vi "Autonomous.vi"(11 "Call Context":T7) -> (0 "SubState 2":T2, 1 "Loop 2 Data":T3, 2 "SubState 1":T2, 3 "Loop 1 Data":T4, 4 "Loop 3 Data":T1, 5 "SubState 0":T2=enum."driver control", 6 "SubState 3":T2, 7 "Loop 0 Data":T5, 10 "SubState 4":T6)   [LabVIEW 2013]
uses:
  typedefs/State Machine/subStates.ctl
  <vilib>/Rock Robotics/WPI/DriverStation/WPI_DriverStationDerivedRobotMode.ctl
  typedefs/State Machine/singleUseSubstate.ctl
  typedefs/Loop Datatypes/Loop 0 Datatype.ctl
  typedefs/Loop Datatypes/Loop 1 Datatype.ctl
  typedefs/Loop Datatypes/Loop 2 Datatype.ctl
  typedefs/Loop Datatypes/Loop 3 Datatype.ctl
  typedefs/Vision/vision enable.ctl
  typedefs/fg_typedef.ctl
panel:
  # "Autonomous Loop Data"
  # "Robot Drive"
  # "State Machine Master"
  # "Pickup/Passing Belts"
  # "Pickup/Passing Arm"
  # "Pneumatics"
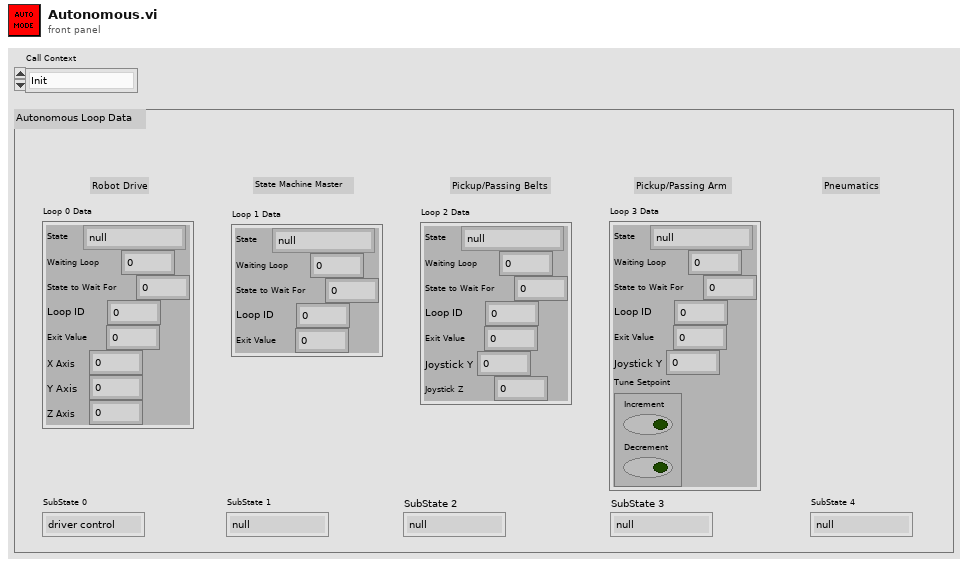
[diagram p1: front panel]
types:
  T1 = typedef "Loop 3 Datatype.ctl" = cluster{"State":T2, "Waiting Loop":i32, "State to Wait For":i32, "Loop ID":i32, "Exit Value":i32, "Joystick Y":dbl, "Tune Setpoint":cluster{"Increment":bool, "Decrement":bool}}
  T2 = typedef "subStates.ctl" = enum16{"null", "wait", "driver control", "auto", "manual override", "hold position", "rotate", "pickup", "pass", "recover pass", "load", "goto shoot", "shoot high goal", "shoot low goal", "cancel arm", "cancel shooter", "end", "test"}
  T3 = typedef "Loop 2 Datatype.ctl" = cluster{"State":T2, "Waiting Loop":i32, "State to Wait For":i32, "Loop ID":i32, "Exit Value":i32, "Joystick Y":dbl, "Joystick Z":dbl}
  T4 = typedef "Loop 1 Datatype.ctl" = cluster{"State":T2, "Waiting Loop":i32, "State to Wait For":i32, "Loop ID":i32, "Exit Value":i32}
  T5 = typedef "Loop 0 Datatype.ctl" = cluster{"State":T2, "Waiting Loop":i32, "State to Wait For":i32, "Loop ID":i32, "Exit Value":i32, "X Axis":dbl, "Y Axis":dbl, "Z Axis":dbl}
  T6 = typedef "singleUseSubstate.ctl" = enum16{"null", "wait", "shift high", "shift low", "extend shooter", "retract shooter", "latch", "unlatch", "end"}
  T7 = typedef "WPI_DriverStationDerivedRobotMode.ctl" = enum16{"Init", "Execute", "Stop"}
  T8 = typedef "fg_typedef.ctl" = enum16{"Get", "Set"}
  T9 = typedef "vision enable.ctl" = enum16{"Enable", "Disable", "Stop"}
  T10 = typedef "WPI_EncoderDevRef.ctl" = cluster{"DevStatus":errorcluster, "EncoderIndex":T11, "CounterIndex":T12, "DistancePerCount":dbl, "Decoding Type":T13}
  T11 = typedef "FPGA_EncoderIdx.ctl" = enum8{"Enc 0", "Enc 1", "Enc 2", "Enc 3", "Invalid"}
  T12 = typedef "FPGA_CounterCtrSystemIndex.ctl" = enum8{"Ctr 0", "Ctr 1", "Ctr 2", "Ctr 3", "Ctr 4", "Ctr 5", "Ctr 6", "Ctr 7", "Invalid"}
  T13 = typedef "WPI_EncoderType.ctl" = enum16{"1x", "2x", "4x"}
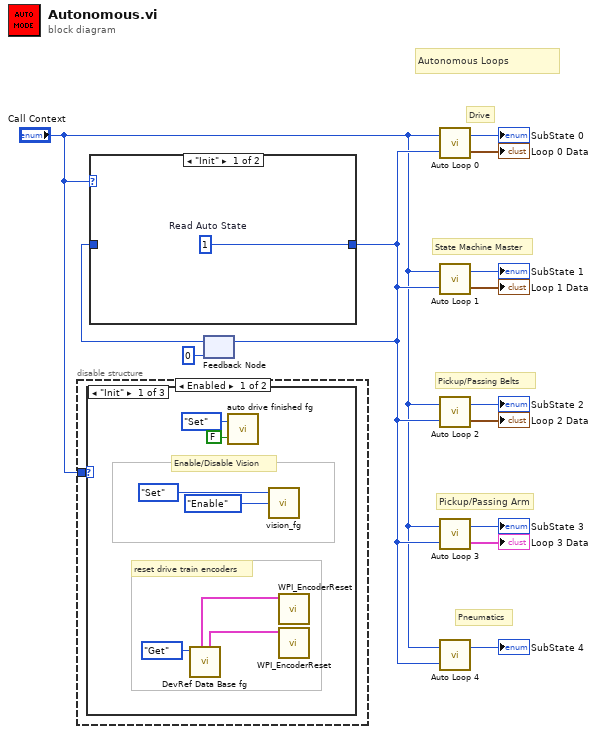
[diagram p0: block diagram]
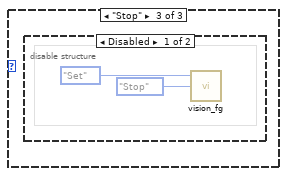
[diagram p3: hidden frame]
diagram:
  # "Autonomous Loops"
  # "Pickup/Passing Arm"
  # "Pickup/Passing Belts"
  # "Pneumatics"
  # "State Machine Master"
  # "Drive"
  n1 = disable-structure shown="Enabled" {
    disable-tunnel: "Call Context" -> [w14 _]
    frame Enabled {
      n2 = case shown="\"Init\"" w14 {
        frame "Init" {
          # "Enable/Disable Vision"
          # "reset drive train encoders"
          n3 = call "DevRef Data Base fg.vi"("Menu"=fg_typedef."Get") -> ("right drive encoder"=w17:T10, "left drive encoder"=w18:T10)  [unwired: 2 in, 7 out]
          n4 = call "auto drive finished fg.vi"("Done?"=FALSE, "Menu"=fg_typedef."Set") -> ()  [unwired: 1 out]
          n5 = call "vision_fg.vi"("Action"=vision_enable."Enable", "Menu"=fg_typedef."Set") -> ()  [unwired: 1 in, 2 out]
          n6 = call <vilib>:"WPI_EncoderReset.vi"("EncoderDevRef"=w18) -> ()  [unwired: 9 in, 2 out]
          n7 = call <vilib>:"WPI_EncoderReset.vi"("EncoderDevRef"=w17) -> ()  [unwired: 9 in, 2 out]
        }
        frame "Execute", Default {
        }
        frame "Stop" {
          n8 = disable-structure shown="Disabled" {
            frame Disabled {
              n9 = call "vision_fg.vi"("Action"=vision_enable."Stop", "Menu"=fg_typedef."Set") -> ()  [unwired: 1 in, 2 out]
            }
            frame Enabled {
            }
          }
        }
      }
    }
    frame Disabled {
    }
  }
  n10 = feedback #1(u8 0 ("Read Auto State")) -> (w2:u8)
  n11 = case shown="\"Init\"" "Call Context" {
    tunnel: [w24 w25] -> w4
    tunnel: w2 -> [_ w25]
    frame "Init" {
      w24 = u8 1  # Read Auto State
    }
    frame "Execute", Default {
    }
  }
  n12 = feedback-in #1(w4) -> ()
  n13 = call "Auto Loop 0.vi"("Auto State"=w4, "Call Context"="Call Context") -> ("Loop 0 Data"=→"Loop 0 Data":T5, "SubState 0"=→"SubState 0":T2)
  n14 = call "Auto Loop 1.vi"("Auto State"=w4, "Call Context"="Call Context") -> ("Loop 1 Data"=→"Loop 1 Data":T4, "SubState 1"=→"SubState 1":T2)
  n15 = call "Auto Loop 2.vi"("Auto State"=w4, "Call Context"="Call Context") -> ("Loop 2 Data"=→"Loop 2 Data":T3, "SubState 2"=→"SubState 2":T2)
  n16 = call "Auto Loop 3.vi"("Auto State"=w4, "Call Context"="Call Context") -> ("Loop 3 Data"=→"Loop 3 Data":T1, "SubState 3"=→"SubState 3":T2)
  n17 = call "Auto Loop 4.vi"("Auto State"=w4, "Call Context"="Call Context") -> ("SubState 5"=→"SubState 4":T6)  [unwired: 1 in]
